vi "Instrument Settings.vi"() -> ()   [LabVIEW 2020]
uses:
  UI Manager/dialogs/settings/Display Instrument Settings.ctl
  plugin.lvlib
panel:
  in  "Instrument Configuration":T1
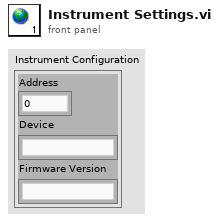
[diagram p1: front panel]
types:
  T1 = typedef "plugin_flodx_ph_probe.lvlib/plugin.lvlib/Display Instrument Settings.ctl" = cluster{"Address":dbl, "Device":string, "Firmware Version":string}
diagram:
